vi "Amplitude To dB.vi"(11 "Amplitude":dbl) -> (3 "dB":dbl)   [LabVIEW 2019, in "Audio Processing.lvlib"]
doc: "Convert the amplitude value into decibels."
uses:
  Audio Processing.lvlib
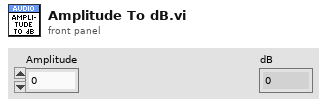
[diagram p1: front panel]
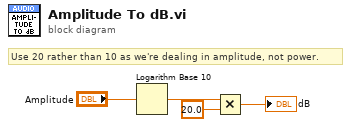
[diagram p0: block diagram]
diagram:
  # "Use 20 rather than 10 as we're dealing in amplitude, not power."
  n1 = Logarithm Base 10(1:"Amplitude") -> (0:w4:dbl)
  n2 = Multiply(x=w4, y=20.0) -> (x*y=→"dB":dbl)
